vi "Parameter 1 Adjust.vi"(0 "Parameter 1 In":T2(ring) caption="Parameter 1", 1 "Previous Parameter 1":T2(ring), 2 "ProgramMode":T1, 5 "Parameter 2 In":enum16{"Voltage", "Pressure", "Flow", "Speed"}(ring)=enum."Pressure" caption="Parameter 2", 7 "Setpoint 2 In":dbl caption="Setpoint 2" min=-1.0 max=800.0, 9 "Setpoint 1 In":dbl caption="Setpoint 1" min=-1.0 max=18.0, 11 "P1 Disabled Items In":i32[](array[numeric])) -> (4 "SP1 Disabled":T3(ring), 6 "Parameter 1 Out":T2(ring), 8 "Parameter 2 Out":T2(ring), 10 "Setpoint 1 Out":dbl, 13 "P2 Disabled Items Out":i32[](array[numeric]), 14 "P1 Disabled Items Out":i32[](array[numeric]), 15 "Setpoint 2 Out":dbl)   [LabVIEW 2013]
uses:
  TypeDef/ProgramMode(PC).ctl
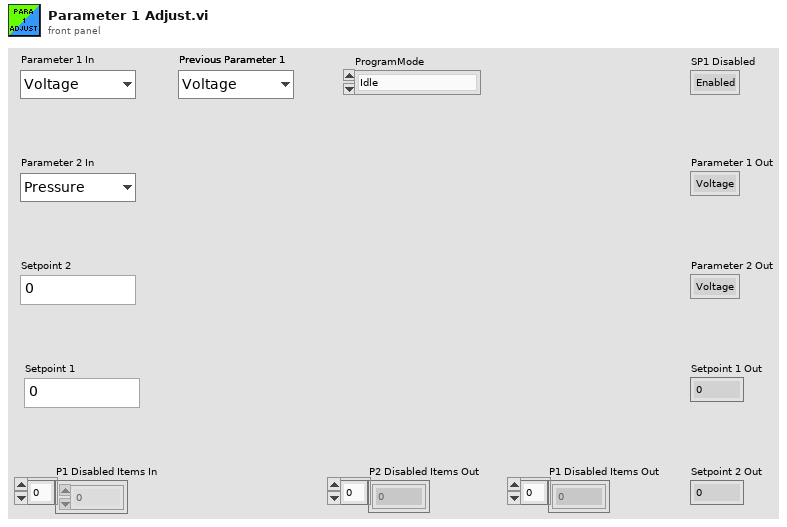
[diagram p1: front panel]
types:
  T1 = typedef "ProgramMode(PC).ctl" = enum16{"Idle", "Manual", "Flow", "Fix Data Point", "Guided Flow", "Timed Test", "Hot Fuel"}
  T2 = enum16{"Voltage", "Pressure", "Flow", "Speed", "Deadhead"}
  T3 = enum8{"Enabled", "Disabled", "Disabled and Grayed Out"}
  T4 = enum16{"Voltage", "Pressure", "Flow", "Speed", "Deadhead"}[]
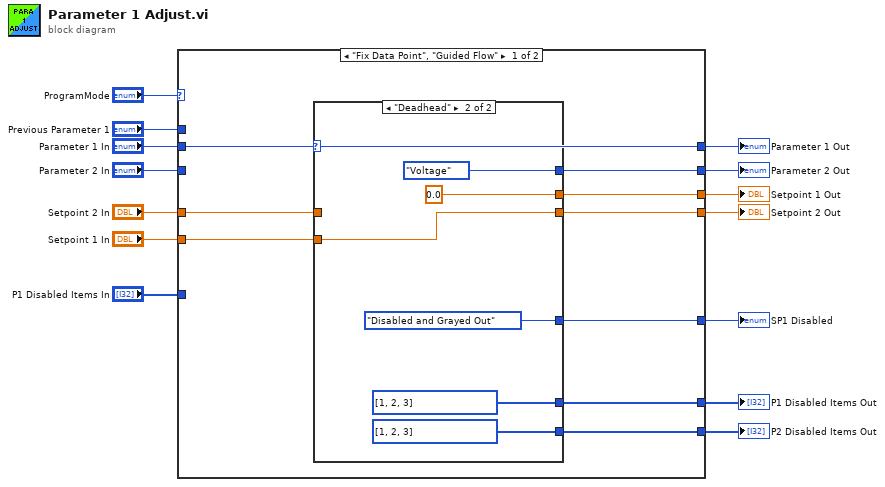
[diagram p0: block diagram]
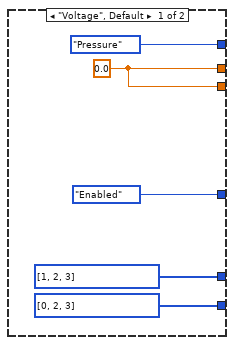
[diagram p2: hidden frame]
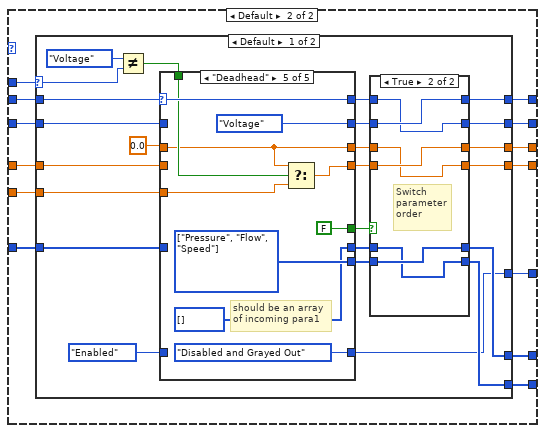
[diagram p3: hidden frame]
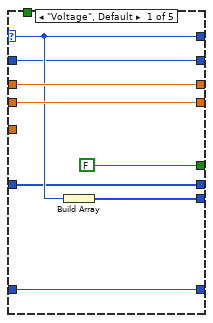
[diagram p5: hidden frame]
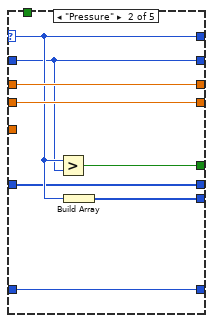
[diagram p6: hidden frame]
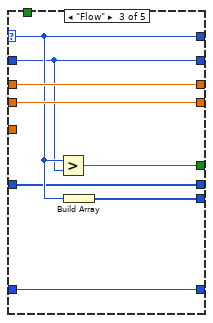
[diagram p7: hidden frame]
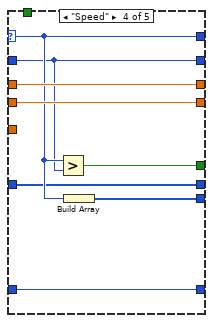
[diagram p8: hidden frame]
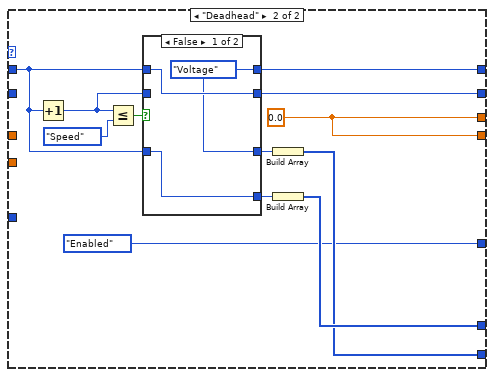
[diagram p9: hidden frame]
diagram:
  n1 = case shown="\"Fix Data Point\", \"Guided Flow\"" "ProgramMode" {
    tunnel: "Parameter 1 In" -> [w22 w47]
    tunnel: [w17 w46] -> w13
    tunnel: "Parameter 2 In" -> [_ w45]
    tunnel: "Setpoint 2 In" -> [w20 w44]
    tunnel: "Setpoint 1 In" -> [w21 w43]
    tunnel: [w22 w42] -> w9
    tunnel: [w23 w41] -> w8
    tunnel: [w19 w40] -> w7
    tunnel: [w18 w39] -> w6
    tunnel: [w15 w38] -> w5
    tunnel: [w16 w37] -> w4
    tunnel: "P1 Disabled Items In" -> [_ w36]
    tunnel: "Previous Parameter 1" -> [_ w35]
    frame "Fix Data Point", "Guided Flow" {
      n2 = case shown="\"Deadhead\"" w22 {
        tunnel: [T2."Pressure" ("Parameter 1 In") T2."Voltage" ("Parameter 1 In")] -> w23
        tunnel: w21 -> [_ w33]
        tunnel: w20 -> [_ _]
        tunnel: [w27 0.0] -> w19
        tunnel: [w27 w33] -> w18
        tunnel: [T3."Enabled" ("Disabled") T3."Disabled and Grayed Out" ("Disabled")] -> w17
        tunnel: [i32[] [0, 2, 3] ("Disabled Items []") i32[] [1, 2, 3] ("Disabled Items []")] -> w16
        tunnel: [i32[] [1, 2, 3] ("Disabled Items []") i32[] [1, 2, 3] ("Disabled Items []")] -> w15
        frame "Voltage", Default {
          w27 = 0.0
        }
        frame "Deadhead" {
        }
      }
    }
    frame Default {
      n3 = case shown="Default" w35 {
        selector: w35 -> [w55 _]
        tunnel: [w69 w135] -> w42
        tunnel: [w68 w127] -> w40
        tunnel: [w67 w133] -> w41
        tunnel: [w66 w127] -> w39
        tunnel: w47 -> [w53 w131]
        tunnel: [w60 w129] -> w38
        tunnel: [w59 w128] -> w37
        tunnel: [w52 T3."Enabled" ("Disabled")] -> w46
        tunnel: w45 -> [w51 _]
        tunnel: w44 -> [w50 _]
        tunnel: w36 -> [w49 _]
        tunnel: w43 -> [w48 _]
        frame Default {
          n4 = Not Equal?(x=T2."Voltage" ("OldVal"), y=w55) -> (x != y?=w54:bool)
          n5 = case shown="\"Deadhead\"" w53 {
            selector: w53 -> [w87 w95 w103 w111 w123]
            tunnel: w51 -> [w86 w94 w102 w110 _]
            tunnel: [FALSE w99 w107 w115 FALSE] -> w71
            tunnel: 0.0 ("Setpoint1") -> [w88 w97 w105 w113 w118]
            tunnel: [w90 w98 w106 w114 T3."Disabled and Grayed Out" ("Disabled")] -> w52
            tunnel: T3."Enabled" ("Disabled") -> [w90 w98 w106 w114 _]
            tunnel: [w88 w97 w105 w113 w118] -> w64
            tunnel: [w89 w96 w104 w112 w117] -> w63
            tunnel: w50 -> [w89 w96 w104 w112 _]
            tunnel: [w87 w95 w103 w111 w123] -> w62
            tunnel: [w86 w94 w102 w110 enum16{"Voltage", "Pressure", "Flow", "Speed"}."Voltage" ("Parameter2")] -> w61
            tunnel: [w85 w93 w101 w109 w121] -> w58
            tunnel: [w84 w92 w100 w108 i32[] [] ("Disabled Items []")] -> w57
            tunnel: w49 -> [w84 w92 w100 w108 _]
            tunnel: w54 -> [_ _ _ _ w119]
            tunnel: w48 -> [_ _ _ _ w116]
            frame "Voltage", Default {
              n6 = Build Array(w87) -> (w85:T4)
            }
            frame "Pressure" {
              n7 = Greater?(x=w95, y=w94) -> (0:w99:bool)
              n8 = Build Array(w95) -> (w93:T4)
            }
            frame "Flow" {
              n9 = Greater?(x=w103, y=w102) -> (0:w107:bool)
              n10 = Build Array(w103) -> (w101:T4)
            }
            frame "Speed" {
              n11 = Greater?(x=w111, y=w110) -> (0:w115:bool)
              n12 = Build Array(w111) -> (w109:T4)
            }
            frame "Deadhead" {
              w121 = enum16{"Voltage", "Pressure", "Flow", "Speed"}[] [enum."Pressure", enum."Flow", enum."Speed"] items=["Voltage", "Pressure", "Flow", "Speed"]
              # "should be an array\nof incoming para1"
              n13 = Select(t=w118, s=w119, f=w116) -> (s? t:f=w117:dbl)
            }
          }
          n14 = case shown="True" w71 {
            tunnel: [w75 w82] -> w69
            tunnel: [w74 w79] -> w67
            tunnel: [w77 w83] -> w68
            tunnel: [w76 w78] -> w66
            tunnel: w64 -> [w77 w78]
            tunnel: w63 -> [w76 w83]
            tunnel: w62 -> [w75 w79]
            tunnel: w61 -> [w74 w82]
            tunnel: [w72 w81] -> w60
            tunnel: [w73 w80] -> w59
            tunnel: w58 -> [w73 w81]
            tunnel: w57 -> [w72 w80]
            frame False {
              # "Parameters\nare in the\ncorrect order"
            }
            frame True {
              # "Switch\nparameter\norder"
            }
          }
        }
        frame "Deadhead" {
          w127 = 0.0 ("Setpoint1")
          n15 = Increment(x=w131) -> (x+1=w134:T2)
          n16 = Less Or Equal?(x=w134, y=T2."Speed") -> (x <= y?=w136:bool)
          n17 = case shown="False" w136 {
            tunnel: w131 -> [w139 w143]
            tunnel: [w138 w143] -> w135
            tunnel: w131 -> [w140 w142]
            tunnel: [w138 w142] -> w130
            tunnel: w134 -> [_ w141]
            tunnel: [w139 w141] -> w133
            tunnel: [w140 w141] -> w132
            frame False {
              w138 = T2."Voltage" ("NewVal")
            }
            frame True {
            }
          }
          n18 = Build Array(w130) -> (w128:T4)
          n19 = Build Array(w132) -> (w129:T4)
        }
      }
    }
  }
  "Parameter 1 Out" <- w9
  "Parameter 2 Out" <- w8
  "Setpoint 1 Out" <- w7
  "Setpoint 2 Out" <- w6
  "P1 Disabled Items Out" <- w5
  "P2 Disabled Items Out" <- w4
  "SP1 Disabled" <- w13
